vi "Get_requested_rows_from_files.vi"(3 "Last File":bool, 4 "First file":bool, 5 "Filename":path, 6 "Selected Rows":i32[](array[numeric])) -> ()   [LabVIEW 2014]
uses:
  Globals/Constants_global.vi
panel:
  out "Ch names Out":string[](array[string])
  out "Channel Values Out":string[][](array[string])
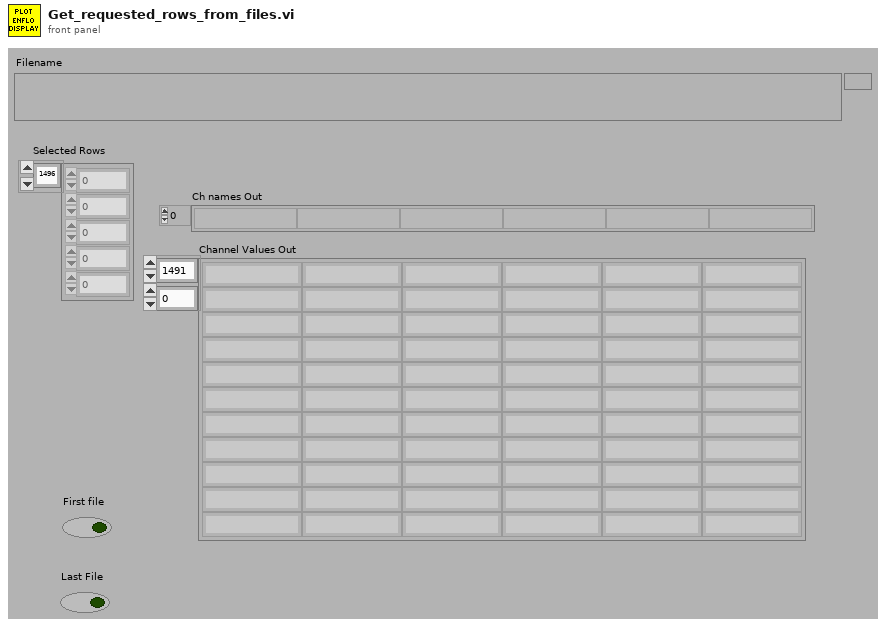
[diagram p1: front panel]
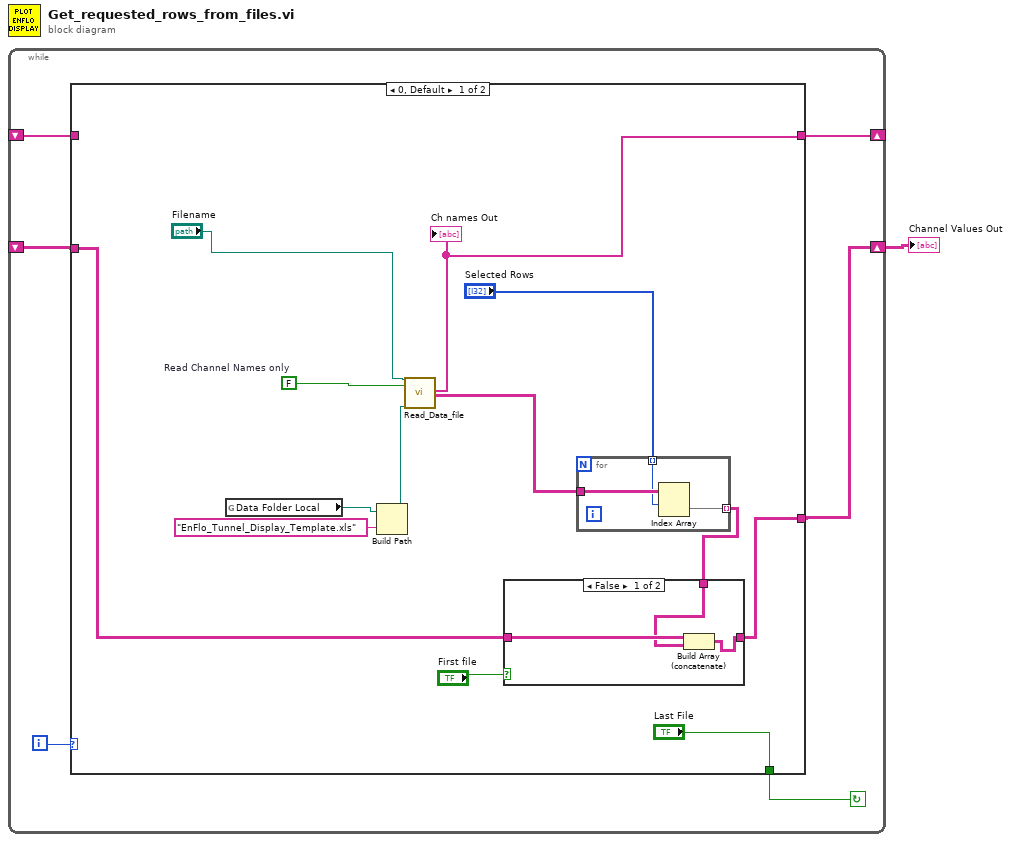
[diagram p0: block diagram]
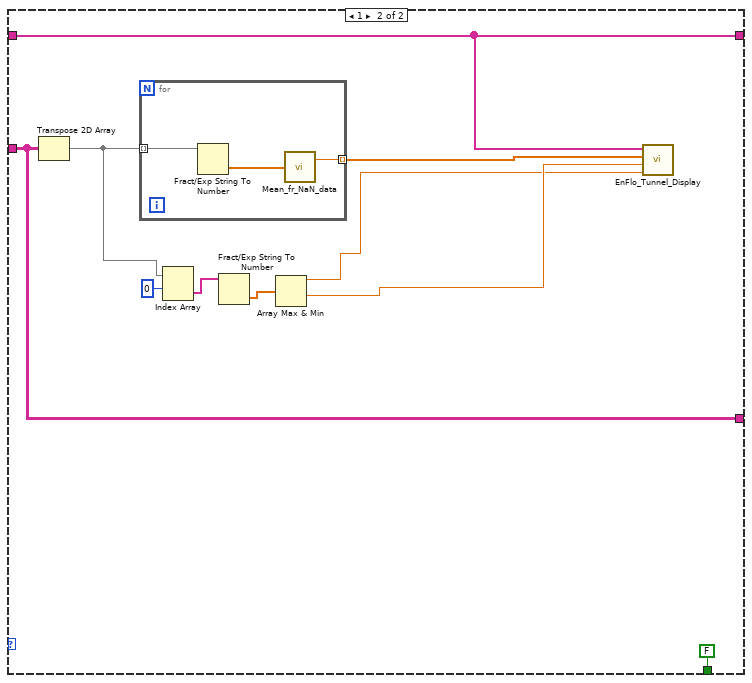
[diagram p3: hidden frame]
diagram:
  n1 = while {
    shift-right: [w6] -> w1
    shift-left: _ -> [w7]
    shift-right: [w4] -> _
    shift-left: _ -> [w3]
    i -> [w2]
    stop <- w5 continue-if-true
    n2 = case shown="0, Default" w2 {
      tunnel: [w12 w35] -> w6
      tunnel: w7 -> [w11 w35]
      tunnel: ["Last File" FALSE ("Last File")] -> w5
      tunnel: [w9 w36] -> w4
      tunnel: w3 -> [_ w36]
      frame 0, Default {
        w16 = FALSE  # Read Channel Names only
        n3 = global read "Constants_global.vi" "Data Folder Local"() -> (w18:path)
        n4 = Build Path(base path=w18, name or relative path="EnFlo_Tunnel_Display_Template.xls") -> (appended path=w19:path)
        n5 = call "Read_Data_file.vi"("Results file"="Filename", "Read Channel Names only"=w16, "Template File"=w19) -> ("Ch names Out"=w9:string[], "Channel Values Out"=w20:string[][])  [unwired: 2 in, 13 out]
        "Ch names Out" <- w9
        n6 = for {
          tunnel: w20 -> [w27]
          tunnel: "Selected Rows" -> [w26] mode=indexing
          tunnel: [w25] -> w13 mode=indexing
          n7 = Index Array(array=w27, index (row)=w26) -> (element=w25:string[])  [unwired: 1 in]
        }
        n8 = case shown="False" "First file" {
          tunnel: [w21 w24] -> w12
          tunnel: w13 -> [w22 w24]
          tunnel: w11 -> [w23 _]
          frame False {
            n9 = Build Array (concatenate)(w23, w22) -> (w21:string[][])
          }
          frame True {
          }
        }
      }
      frame 1 {
        n10 = Transpose 2D Array(2D array=w35) -> (transposed array=w33:string[][])
        n11 = for {
          tunnel: w33 -> [w40] mode=indexing
          tunnel: [w39] -> w37 mode=indexing
          n12 = Fract/Exp String To Number(string=w40) -> (number=w38:dbl[])  [unwired: 3 in, 1 out]
          n13 = call "Mean_fr_NaN_data.vi"("Data"=w38) -> ("Mean value"=w39:dbl)  [unwired: 1 out]
        }
        n14 = Index Array(array=w33, index (row)=0) -> (element=w31:string[])  [unwired: 1 in]
        n15 = Fract/Exp String To Number(string=w31) -> (number=w30:dbl[])  [unwired: 3 in, 1 out]
        n16 = Array Max & Min(array=w30) -> (max value=w28:dbl, min value=w29:dbl)  [unwired: 2 out]
        n17 = call "EnFlo_Tunnel_Display.vi"("End Time"=w28, "Start Time"=w29, "Channel Values"=w37, "Ch names"=w36) -> ()  [unwired: 4 in]
      }
    }
  }
  "Channel Values Out" <- w1
